vi "Dictionary to XY Graph.vi"(8 "error in (no error)":errorcluster, 11 "Results (Dictionary)":cluster{"key":string, "value":dbl}[](array[cluster])) -> (0 "error out":errorcluster, 2 "XY Graph":cluster{dbl[], dbl[]}[](array[cluster]), 3 "Results (Dictionary) out":cluster{"key":string, "value":dbl}[](array[cluster]))   [LabVIEW 2019, in "Instrument UI.Lockin.lvclass"]
uses:
  Instrument.Lockin/Typedefs/Results Type--Enum.ctl
  Instrument UI.Lockin.lvclass
  Instrument.Lockin/Instrument.Lockin.lvclass
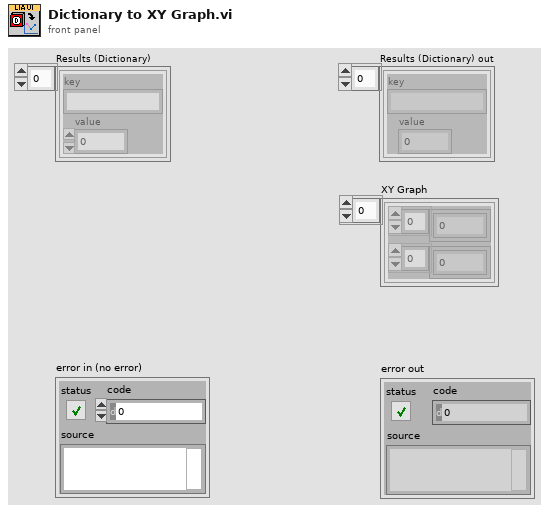
[diagram p1: front panel]
types:
  T1 = typedef "Instrument.Lockin.lvclass/Results Type--Enum.ctl" = enum16{"X", "Y", "R", "Theta", "Mean"}
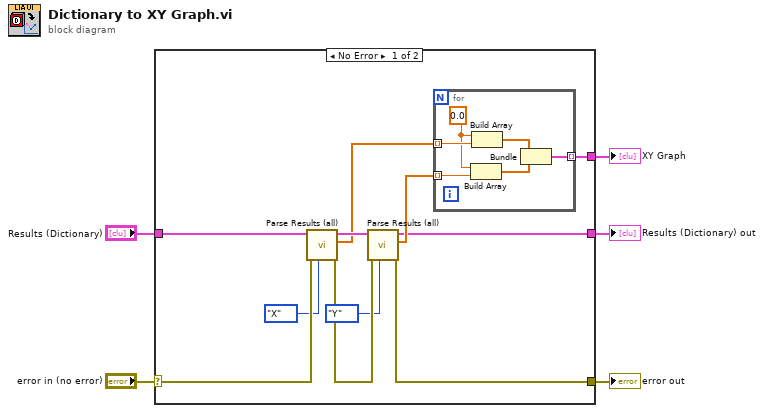
[diagram p0: block diagram]
diagram:
  n1 = case shown="No Error" "error in (no error)" {
    selector: "error in (no error)" -> [w14 w23]
    tunnel: "Results (Dictionary)" -> [w15 _]
    tunnel: [w11 w23] -> w3
    tunnel: [w16 _] -> w2
    tunnel: [w6 _] -> w1
    frame No Error {
      n2 = call "Parse Results (all).vi"("Type"=Results_Type--Enum."X", "error in (no error)"=w14, "Results (Dictionary)"=w15) -> ("error out"=w12:errorcluster, "Data"=w7:dbl[], "Results (Dictionary)"=w13:cluster{"key":string, "value":dbl}[])  [unwired: 5 in, 1 out]
      n3 = call "Parse Results (all).vi"("Type"=Results_Type--Enum."Y", "error in (no error)"=w12, "Results (Dictionary)"=w13) -> ("error out"=w11:errorcluster, "Data"=w8:dbl[], "Results (Dictionary)"=w6:cluster{"key":string, "value":dbl}[])  [unwired: 5 in, 1 out]
      n4 = for {
        tunnel: w7 -> [w22] mode=indexing
        tunnel: w8 -> [w21] mode=indexing
        tunnel: [w17] -> w16 mode=indexing
        w20 = 0.0
        n5 = Build Array(w20, w21) -> (w18:dbl[])
        n6 = Build Array(w20, w22) -> (w19:dbl[])
        n7 = Bundle(w19, w18) -> (w17:cluster{dbl[], dbl[]})  [unwired: 1 in]
      }
    }
    frame Error {
    }
  }
  "error out" <- w3
  "XY Graph" <- w2
  "Results (Dictionary) out" <- w1
